vi "ocdemo.vi"() -> ()   [LabVIEW 2012]
panel:
  out "U8":u8[](array[numeric])
  in  "布尔":bool
  in  "停止":bool
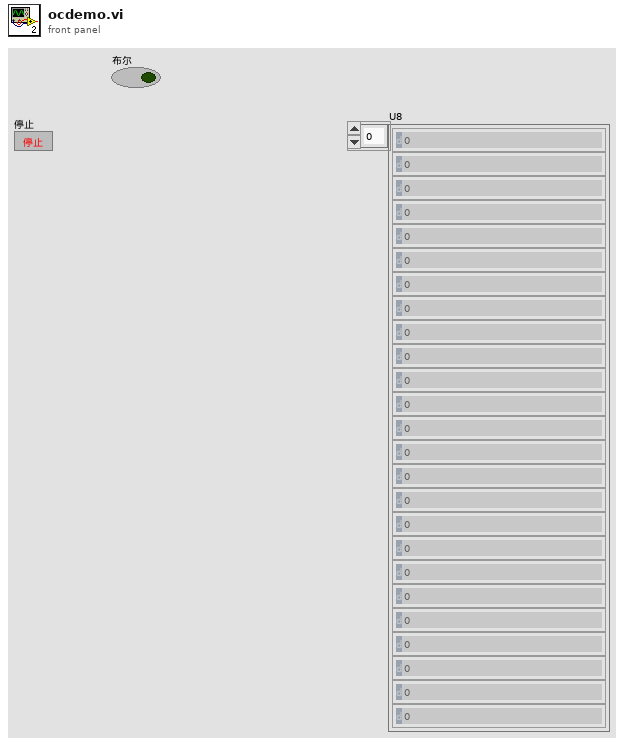
[diagram p1: front panel]
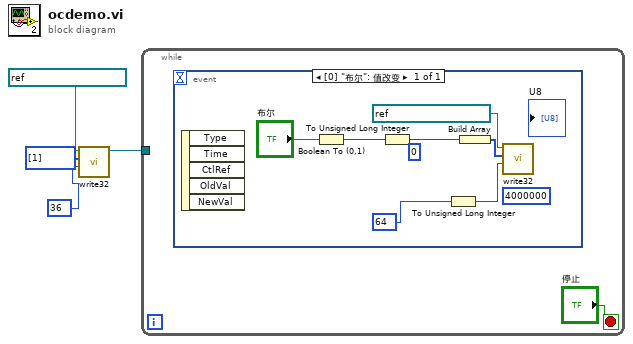
[diagram p0: block diagram]
diagram:
  n1 = call "write32.vi"("起始地址"=36 ("x"), "U32"=u32[] [1], "VISA资源名称输入"=refnum<visa-resource-name> "PXI1::12::INSTR") -> ("VISA资源名称输出"=w1:refnum<visa-resource-name>)  [unwired: 7 in, 1 out]
  n2 = while {
    tunnel: w1 -> [_]
    stop <- "停止" stop-if-true
    n3 = event shown="[0] \"布尔\": 值改变" {
      selector: _ -> [_]
      dyn-events: _ -> [_]
      timeout: _ -> [_]
      event "布尔": Value Change {
        (unwired) u32 4000000 ("元素")
        (unwired) u32 0 ("元素")
        n4 = event-data() -> ()  [unwired: 1 in, 5 out]
        n5 = Boolean To (0,1)(Boolean="布尔") -> (0, 1=w12:i16)
        n6 = To Unsigned Long Integer(number=w12) -> (unsigned 32bit integer=w10:u32)
        n7 = To Unsigned Long Integer(number=64 ("x")) -> (unsigned 32bit integer=w9:u32)
        n8 = Build Array(w10) -> (w8:u32[])
        n9 = call "write32.vi"("起始地址"=w9, "U32"=w8, "VISA资源名称输入"=refnum<visa-resource-name> "PXI1::12::INSTR") -> ()  [unwired: 7 in, 2 out]
      }
    }
  }
